vi "AWG_5421_Run_Async.vi"(8 "error in (no error)":errorcluster, 10 "Use Software trigger":bool, 11 "AWG5421 Resource Name":refnum<k15>) -> (0 "error out":errorcluster)   [LabVIEW 2017]
doc: "This VI runs asynchronously. It starts a waveform generation in response to one or many triggers, and waits until the end of the generation before to stop."
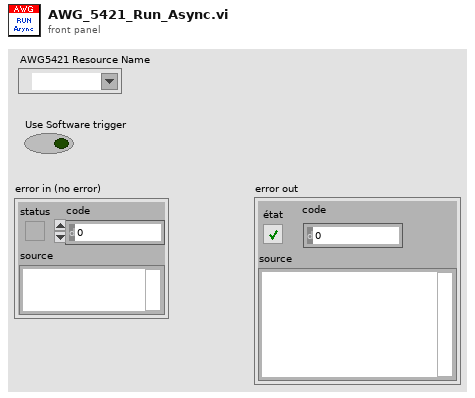
[diagram p1: front panel]
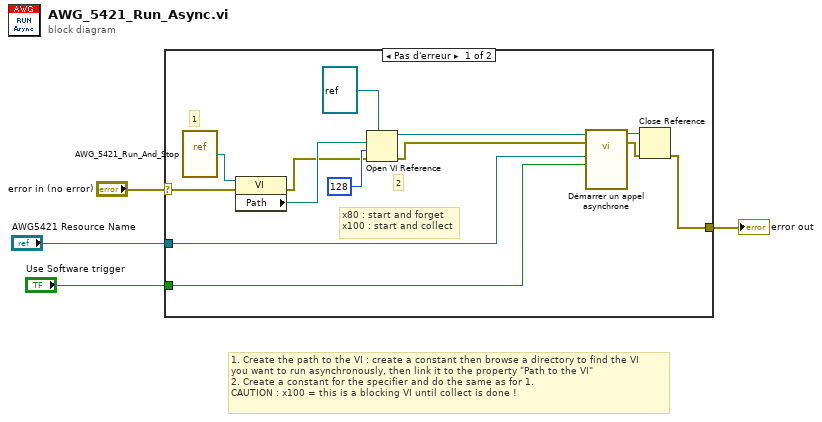
[diagram p0: block diagram]
diagram:
  # "1. Create the path to the VI : create a constant then browse a directory to find the VI\nyou want to run asynchronously, then link it to the property \"Path to the VI\"\n2. Create a constant for the specifier and do the same as for 1.\nCAUTION : x100 = this is a blocking VI until collect is done !"
  n1 = case shown="Pas d'erreur" "error in (no error)" {
    selector: "error in (no error)" -> [w15 w18]
    tunnel: [w5 w18] -> w3
    tunnel: "AWG5421 Resource Name" -> [w13 _]
    tunnel: "Use Software trigger" -> [w12 _]
    frame No Error {
      # "1"
      # "2"
      # "x80 : start and forget\nx100 : start and collect"
      n2 = vi-ref "AWG_5421_Run_And_Stop.vi"() -> (w8:refnum<vi>)
      n3 = property class="VI"(reference=w8, error in=w15) -> (error out=w14:errorcluster, "Path"=w16:path)  [unwired: 1 out]
      n4 = Open VI Reference(type specifier VI Refnum (for type only)=refnum<vi> refnum ("spécificateur de type du refnum de VI (pour type seulement)"), vi path=w16, options=128, error in (no error)=w14) -> (vi reference=w9:refnum<vi>, error out=w11:errorcluster)  [unwired: 2 in]
      n5 = call-by-ref "Démarrer un appel asynchrone"(reference=w9, error in=w11, "Use Software trigger"=w12, "instrument handle in"=w13) -> (reference out=w6:refnum<vi>, error out=w7:errorcluster)  [unwired: 9 in, 1 out]
      n6 = Close Reference(reference=w6, error in (no error)=w7) -> (error out=w5:errorcluster)
    }
    frame Error {
    }
  }
  "error out" <- w3
